vi "Broadcasting Main.vi"(8 "Error In":errorcluster, 11 "Device Connector in":refnum<class "Device Connector.lvclass">) -> (0 "error out (no error)":T1, 3 "Device Connector out":refnum<class "Device Connector.lvclass">)   [LabVIEW 2024, in "Device Connector.lvclass"]
uses:
  Device Connector.lvclass
  Device Connector.lvclass/Device Connector.ctl
  Ancestor Class/Actor Assistant/Observer/Observer.lvclass
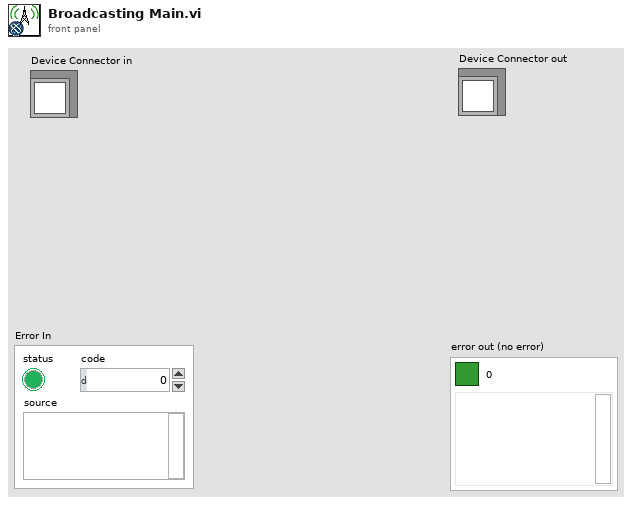
[diagram p1: front panel]
types:
  T1 = cluster{"Boolean Round":bool, "code":i32, "source":string}
  T2 = typedef "Observer Queue.ctl" = refnum<queue>
  T3 = typedef "Stop Observer Loop.ctl" = refnum<notifier>
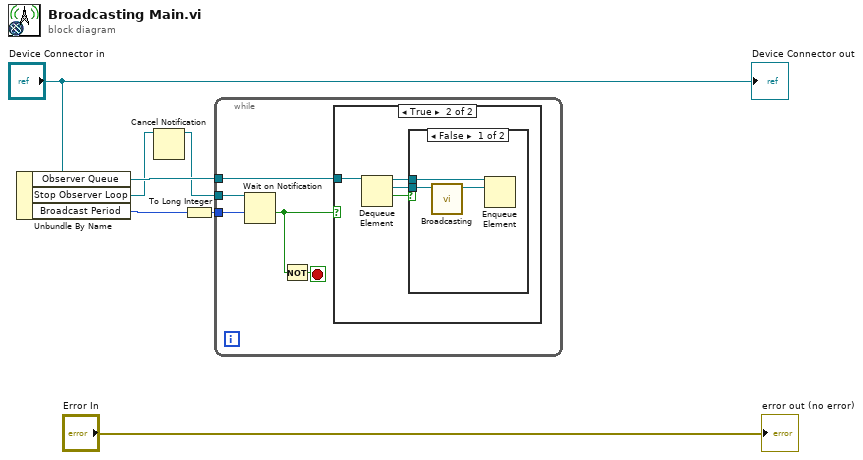
[diagram p0: block diagram]
diagram:
  n1 = Unbundle By Name("Device Connector in") -> ("Observer Queue"=w3:T2, "Stop Observer Loop"=w2:T3, "Broadcast Period"=w6:u32)
  n2 = Cancel Notification(0:w2) -> (8:w1:T3)  [unwired: 1 in, 2 out]
  n3 = To Long Integer(number=w6) -> (32bit integer=w5:i32)
  n4 = while {
    tunnel: w5 -> [w12]
    tunnel: w1 -> [w11]
    tunnel: w3 -> [w8]
    stop <- w10 stop-if-true
    n5 = Wait on Notification(notifier=w11, timeout in ms (-1)=w12) -> (timed out?=w9:bool)  [unwired: 2 in, 3 out]
    n6 = Not(x=w9) -> (.not. x?=w10:bool)
    n7 = case shown="True" w9 {
      tunnel: w8 -> [_ w16]
      frame False {
      }
      frame True {
        n8 = Dequeue Element(queue=w16) -> (queue out=w14:T2, element=w15:refnum<class "Observer.lvclass">, timed out?=w13:bool)  [unwired: 2 in, 1 out]
        n9 = case shown="False" w13 {
          tunnel: w15 -> [w19 _]
          tunnel: w14 -> [w18 _]
          frame False {
            n10 = call-dynamic "Broadcasting.vi"("Observer in"=w19) -> ("Observer out"=w17:refnum<class "Observer.lvclass">)  [unwired: 9 in, 1 out]
            n11 = Enqueue Element(queue=w18, element=w17) -> ()  [unwired: 2 in, 3 out]
          }
          frame True {
          }
        }
      }
    }
  }
  "Device Connector out" <- "Device Connector in"
  "error out (no error)" <- "Error In"
